vi "GetRawFolder.vi"(11 "File name":path) -> (3 "Path to Raw data":path)   [LabVIEW 2022 SP3]
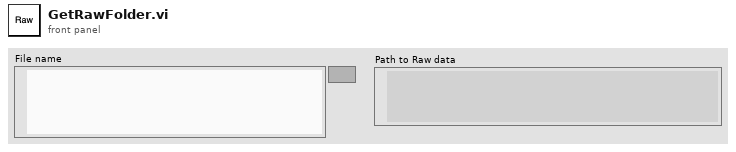
[diagram p1: front panel]
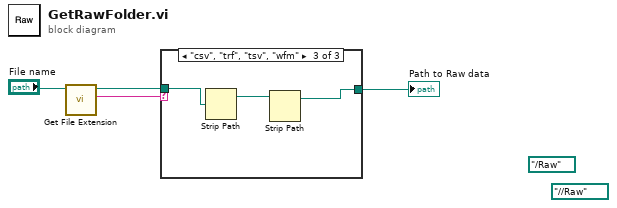
[diagram p0: block diagram]
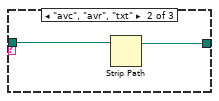
[diagram p3: hidden frame]
diagram:
  (unwired) path "../../Raw" ("name or relative path")
  (unwired) path "../Raw" ("name or relative path")
  n1 = call <vilib>:"Get File Extension.vi"("file"="File name") -> ("lowercase file extension"=w3:string, "dup file"=w4:path)  [unwired: 6 in, 3 out]
  n2 = case shown="\"csv\", \"trf\", \"tsv\", \"wfm\"" w3 {
    tunnel: w4 -> [w5 w7 w10]
    tunnel: [w5 w6 w8] -> w2
    frame Default {
    }
    frame "avc", "avr", "txt" {
      n3 = Strip Path(path=w7) -> (stripped path=w6:path)  [unwired: 1 out]
    }
    frame "csv", "trf", "tsv", "wfm" {
      n4 = Strip Path(path=w10) -> (stripped path=w9:path)  [unwired: 1 out]
      n5 = Strip Path(path=w9) -> (stripped path=w8:path)  [unwired: 1 out]
    }
  }
  "Path to Raw data" <- w2
